vi "json_variant_set_name.vi"(8 "error in (no error)":errorcluster, 10 "name":string, 11 "variant in":variant) -> (0 "error out":errorcluster, 3 "variant out":variant)   [LabVIEW 2017]
uses:
  <vilib>/Utility/Data Type/NI_Data Type.lvlib
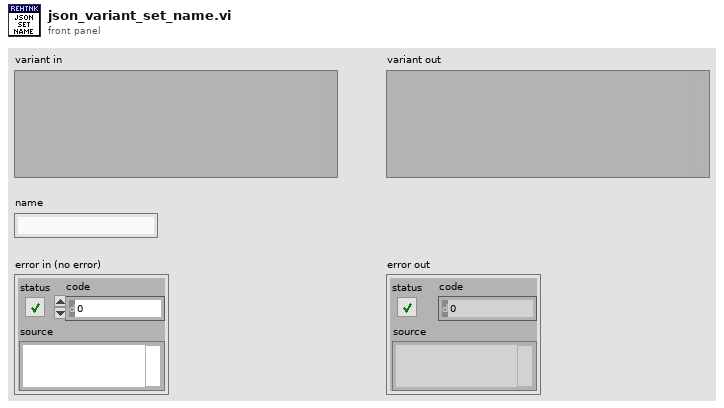
[diagram p1: front panel]
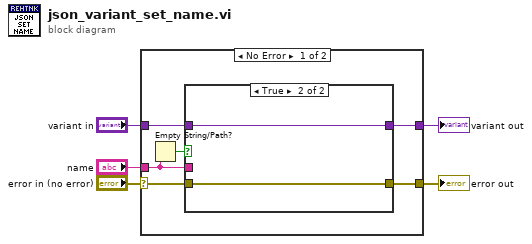
[diagram p0: block diagram]
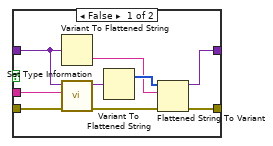
[diagram p2: hidden frame]
diagram:
  n1 = case shown="No Error" "error in (no error)" {
    selector: "error in (no error)" -> [w6 w24]
    tunnel: [w7 w24] -> w5
    tunnel: [w11 w23] -> w3
    tunnel: "variant in" -> [w10 w23]
    tunnel: "name" -> [w9 _]
    frame No Error {
      n2 = Empty String/Path?(string/path=w9) -> (empty?=w8:bool)
      n3 = case shown="True" w8 {
        tunnel: [w13 w22] -> w11
        tunnel: w10 -> [w14 w22]
        tunnel: w9 -> [w12 _]
        tunnel: [w15 w21] -> w7
        tunnel: w6 -> [w16 w21]
        frame False {
          n4 = Variant To Flattened String(Variant=w14) -> (data string=w17:string)  [unwired: 1 out]
          n5 = call <vilib>:"Set Type Information.vi"("error in (no error)"=w16, "Name"=w12, "Variant in"=w14) -> ("error out"=w20:errorcluster, "Variant out"=w19:variant)  [unwired: 7 in]
          n6 = Variant To Flattened String(Variant=w19) -> (1:w18:i16[])  [unwired: 1 out]
          n7 = Flattened String To Variant(4:w20, 6:w17, 7:w18) -> (0:w15:errorcluster, 3:w13:variant)
        }
        frame True {
        }
      }
    }
    frame Error {
    }
  }
  "error out" <- w5
  "variant out" <- w3
